vi "new현재날자(SubVI).vi"() -> (0 "월,일 을 문자열로":string, 1 "월,일 을 숫자열로":i32, 2 "월":i32, 3 "일":i32, 4 "일 문자열":string, 5 "날짜/시간 문자열":string, 6 "월 문자열":string)   [LabVIEW 2014]
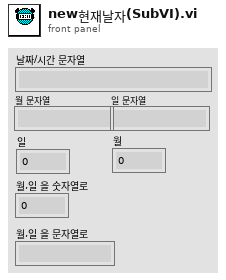
[diagram p1: front panel]
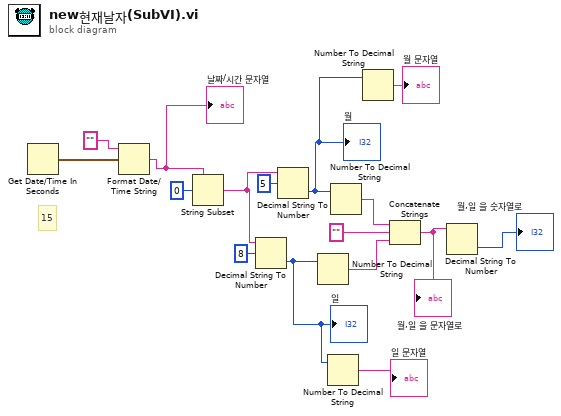
[diagram p0: block diagram]
diagram:
  # "15"
  n1 = Get Date/Time In Seconds() -> (seconds since 1Jan1904=w11:timestamp)
  n2 = Format Date/Time String(time format string (%c)="" ("시간 포맷 문자열 (%c)"), seconds (now)=w11) -> (date/time string=w7:string)  [unwired: 1 in]
  "날짜/시간 문자열" <- w7
  n3 = String Subset(string=w7, offset (0)=0 ("오프셋(0)")) -> (substring=w15:string)  [unwired: 1 in]
  n4 = Decimal String To Number(string=w15, offset=8 ("오프셋")) -> (number=w6:i32)  [unwired: 1 in, 1 out]
  "일" <- w6
  n5 = Decimal String To Number(string=w15, offset=5 ("오프셋")) -> (number=w4:i32)  [unwired: 1 in, 1 out]
  "월" <- w4
  n6 = Number To Decimal String(number=w6) -> (decimal integer string=w2:string)  [unwired: 1 in]
  n7 = Number To Decimal String(number=w6) -> (decimal integer string=→"일 문자열":string)  [unwired: 1 in]
  n8 = Number To Decimal String(number=w4) -> (decimal integer string=w16:string)  [unwired: 1 in]
  n9 = Number To Decimal String(number=w4) -> (decimal integer string=→"월 문자열":string)  [unwired: 1 in]
  n10 = Concatenate Strings(w16, "", w2) -> (w9:string)
  "월,일 을 문자열로" <- w9
  n11 = Decimal String To Number(string=w9) -> (number=→"월,일 을 숫자열로":i32)  [unwired: 2 in, 1 out]
